vi "configure data acquisition.vi"() -> (1 "sampling rate (samples/sec) 2":dbl=1000.0, 2 "samples per acquisition 2":dbl=10000.0)   [LabVIEW 2014]
panel:
  in  "OK Button":bool
  in  "samples per acquisition":dbl=10000.0
  in  "sampling rate (samples/sec)":dbl=1000.0
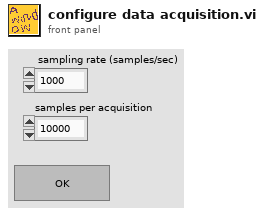
[diagram p1: front panel]
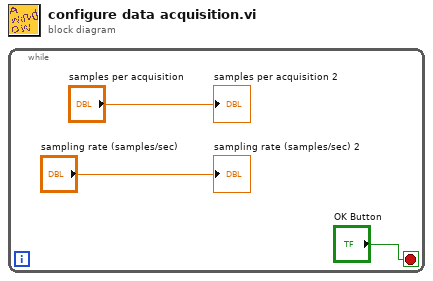
[diagram p0: block diagram]
diagram:
  n1 = while {
    stop <- "OK Button" stop-if-true
    "sampling rate (samples/sec) 2" <- "sampling rate (samples/sec)"
    "samples per acquisition 2" <- "samples per acquisition"
  }
